vi "Simulated_Field_FIELD_ODOM_CLAMP.vi"(11 "in Sim Pose":T1={"TRANSLATION"={"X"=0.0, "Y"=0.0}, "ROTATION"={"VALUE"=0.0, "COS"=1.0, "SIN"=0.0}} {"ROTATION"."SIN" format="%13.4f"; "ROTATION"."COS" format="%13.4f"; "ROTATION"."VALUE" format="%13.4f"; "TRANSLATION"."Y" format="%14.3f"; "TRANSLATION"."X" format="%14.3f"}) -> (3 "out Sim Pose":T1={"TRANSLATION"={"X"=0.0, "Y"=0.0}, "ROTATION"={"VALUE"=0.0, "COS"=1.0, "SIN"=0.0}} {"ROTATION"."SIN" format="%13.4f"; "ROTATION"."COS" format="%13.4f"; "ROTATION"."VALUE" format="%13.4f"; "TRANSLATION"."Y" format="%14.3f"; "TRANSLATION"."X" format="%14.3f"})   [LabVIEW 2019, in "Simulated_Field.lvlib"]
uses:
  <vilib>/Rock Robotics/WPI/ThirdParty/JAS_Junk/TrajLib/TypeDef/POSE2D.ctl
  <vilib>/Rock Robotics/WPI/ThirdParty/JAS_Junk/TrajLib/TypeDef/TRANSLATION2D.ctl
  <vilib>/Rock Robotics/WPI/ThirdParty/JAS_Junk/TrajLib/TypeDef/ROTATION2D.ctl
  Simulated_Field.lvlib
  <vilib>/Rock Robotics/WPI/ThirdParty/JAS_Junk/TrajLib/Trajectory_Library.lvlib
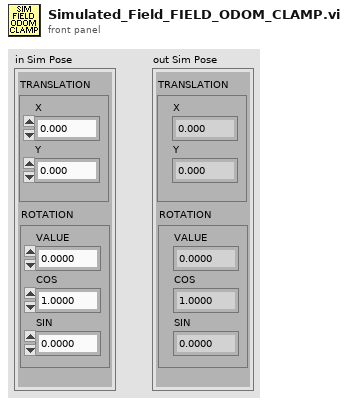
[diagram p1: front panel]
types:
  T1 = typedef "Trajectory_Library.lvlib/POSE2D.ctl" = cluster{"TRANSLATION":T2, "ROTATION":T3}
  T2 = typedef "Trajectory_Library.lvlib/TRANSLATION2D.ctl" = cluster{"X":dbl, "Y":dbl}
  T3 = typedef "Trajectory_Library.lvlib/ROTATION2D.ctl" = cluster{"VALUE":dbl, "COS":dbl, "SIN":dbl}
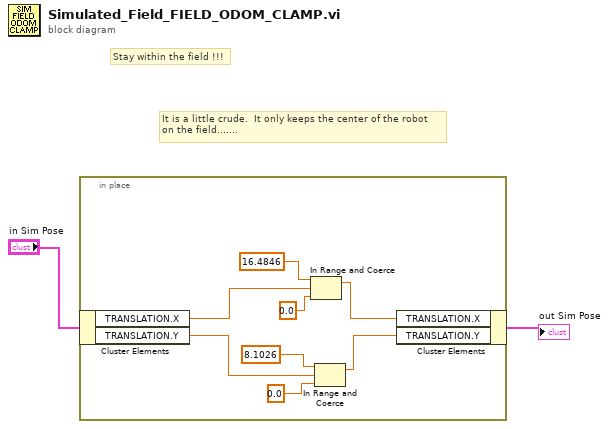
[diagram p0: block diagram]
diagram:
  # "It is a little crude.  It only keeps the center of the robot\non the field......."
  # "Stay within the field !!!"
  n1 = in-place {
    n2 = in-place-cluster #1("in Sim Pose") -> ("TRANSLATION.X"=w8:dbl, "TRANSLATION.Y"=w9:dbl)
    n3 = In Range and Coerce(upper limit=16.4846, x=w8, lower limit=0.0) -> (coerced(x)=w10:dbl)  [unwired: 1 out]
    n4 = In Range and Coerce(upper limit=8.1026, x=w9, lower limit=0.0) -> (coerced(x)=w3:dbl)  [unwired: 1 out]
    n5 = in-place-cluster #1("TRANSLATION.X"=w10, "TRANSLATION.Y"=w3) -> (→"out Sim Pose":T1)
  }
